vi "PositionProfileMove.vi"(7 "Relative?":bool, 8 "error in (no error)":errorcluster, 10 "Array":dbl[](array[numeric]), 11 "SoftmotionAxis in":refnum<class "SoftmotionAxis.lvclass">) -> (0 "error out":errorcluster, 3 "SoftmotionAxis out":refnum<class "SoftmotionAxis.lvclass">)   [LabVIEW 2017, in "SoftmotionAxis.lvclass"]
uses:
  SoftmotionAxis.lvclass
  <resource>/objmgr/nimotion.rc
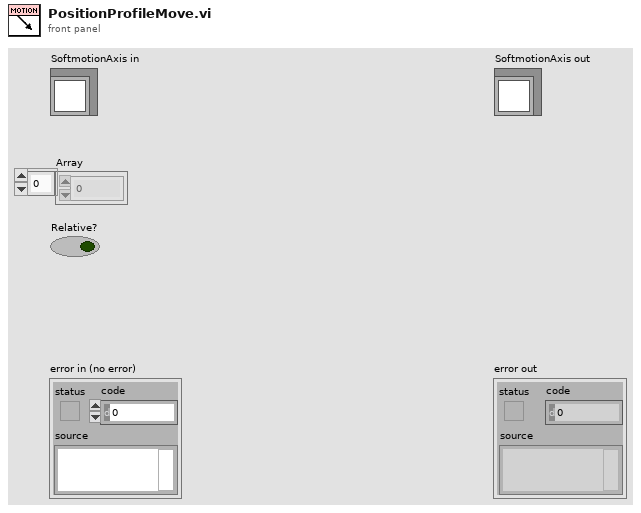
[diagram p1: front panel]
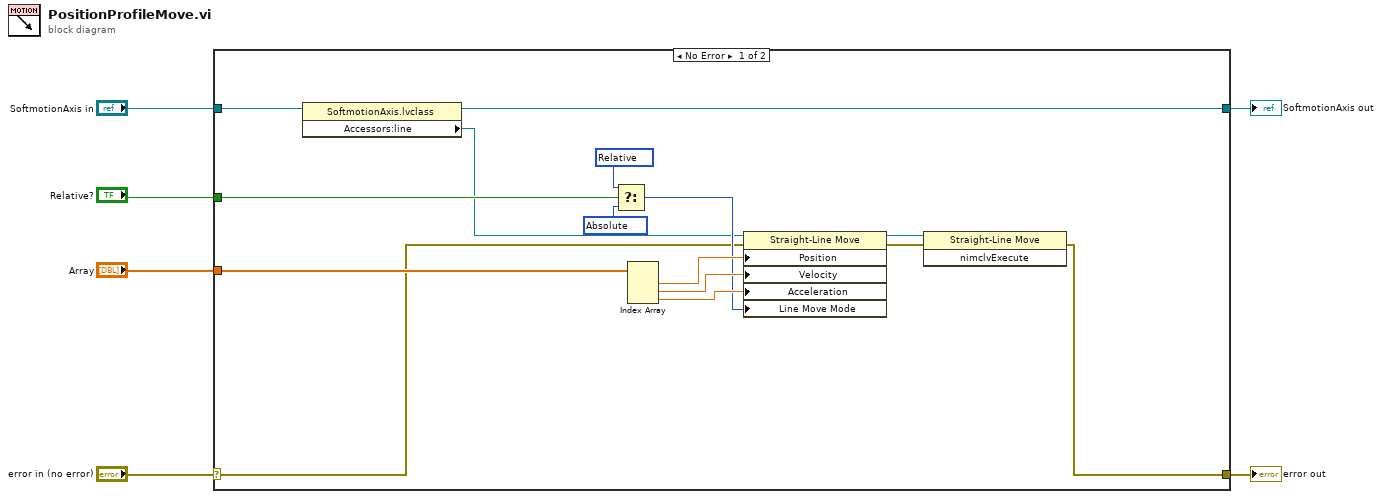
[diagram p0: block diagram]
diagram:
  n1 = case shown="No Error" "error in (no error)" {
    selector: "error in (no error)" -> [w12 w23]
    tunnel: [w11 w23] -> w5
    tunnel: [w8 w22] -> w3
    tunnel: "SoftmotionAxis in" -> [w9 w22]
    tunnel: "Array" -> [w13 _]
    tunnel: "Relative?" -> [w10 _]
    frame No Error {
      w17 = 10551337 items=["Relative"=10551344, "Absolute"=10551337, "Relative To Capture"=10551345, "Velocity"=10551346, "Polyline"=11600101] ("Line Move Mode")
      w18 = 10551344 items=["Relative"=10551344, "Absolute"=10551337, "Relative To Capture"=10551345, "Velocity"=10551346, "Polyline"=11600101] ("Line Move Mode")
      n2 = property class="SoftmotionAxis.lvclass"(reference=w9) -> (reference out=w8:refnum<class "SoftmotionAxis.lvclass">, "Accessors:line"=w7:refnum<k20>)  [unwired: 1 in, 1 out]
      n3 = Select(t=w18, s=w10, f=w17) -> (s? t:f=w16:i32)
      n4 = Index Array(array=w13) -> (element #1=w21:dbl, element #2=w20:dbl, element #3=w19:dbl)  [unwired: 3 in]
      n5 = property class="Straight-Line Move"(reference=w7, error in=w12, "Position"=w21, "Velocity"=w20, "Acceleration"=w19, "Line Move Mode"=w16) -> (reference out=w14:refnum<k20>, error out=w15:errorcluster)
      n6 = invoke class="Straight-Line Move" method="nimclvExecute"(reference=w14, error in=w15) -> (error out=w11:errorcluster)  [unwired: 1 in, 2 out]
    }
    frame Error {
    }
  }
  "error out" <- w5
  "SoftmotionAxis out" <- w3
